vi "Pose2d_NearestTo.vi"(9 "other POSE":T1[](array[typedef]) {"ROTATION"."SIN" format="%13.4f"; "ROTATION"."COS" format="%13.4f"; "ROTATION"."VALUE" format="%13.4f"; "TRANSLATION"."Y" format="%14.3f"; "TRANSLATION"."X" format="%14.3f"}, 11 "in POSE":T1 {"ROTATION"."SIN" format="%13.4f"; "ROTATION"."COS" format="%13.4f"; "ROTATION"."VALUE" format="%13.4f"; "TRANSLATION"."Y" format="%14.3f"; "TRANSLATION"."X" format="%14.3f"}) -> (1 "Found":bool, 3 "Nearest Pose":T1={"TRANSLATION"={"X"=0.0, "Y"=0.0}, "ROTATION"={"VALUE"=0.0, "COS"=1.0, "SIN"=0.0}} {"ROTATION"."SIN" format="%13.4f"; "ROTATION"."COS" format="%13.4f"; "ROTATION"."VALUE" format="%13.4f"; "TRANSLATION"."Y" format="%14.3f"; "TRANSLATION"."X" format="%14.3f"})   [LabVIEW 2019, in "Trajectory_Library.lvlib"]
doc: "Returns the Transform2d that maps the one pose to another.\n\nParameter:\n - IN POSE - Current POSE data structure\n - OTHER POSE - The initial pose of the transformation.\n\nReturns:\n - OUT TRANSFORMATION - The transform that maps the other pose to the current pose."
uses:
  TypeDef/POSE2D.ctl
  TypeDef/TRANSLATION2D.ctl
  TypeDef/ROTATION2D.ctl
  Transform2d_Create_PosePose.vi
  Pose2d_New_TRRO.vi
  Rotation2d_UnaryMinus.vi
  Translation2d_RotateBy.vi
  Translation2d_Minus.vi
  Rotation2d_CreateAngle.vi
  Translation2d_Create.vi
  Rotation2d_RotateBy.vi
  Rotation2d_CreateXY.vi
  Util_CalcDist.vi
  Trajectory_Library.lvlib
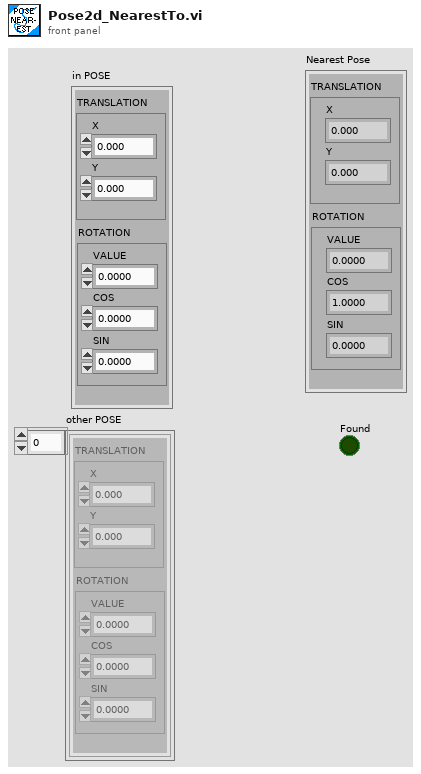
[diagram p1: front panel]
types:
  T1 = typedef "Trajectory_Library.lvlib/POSE2D.ctl" = cluster{"TRANSLATION":T2, "ROTATION":T3}
  T2 = typedef "Trajectory_Library.lvlib/TRANSLATION2D.ctl" = cluster{"X":dbl, "Y":dbl}
  T3 = typedef "Trajectory_Library.lvlib/ROTATION2D.ctl" = cluster{"VALUE":dbl, "COS":dbl, "SIN":dbl}
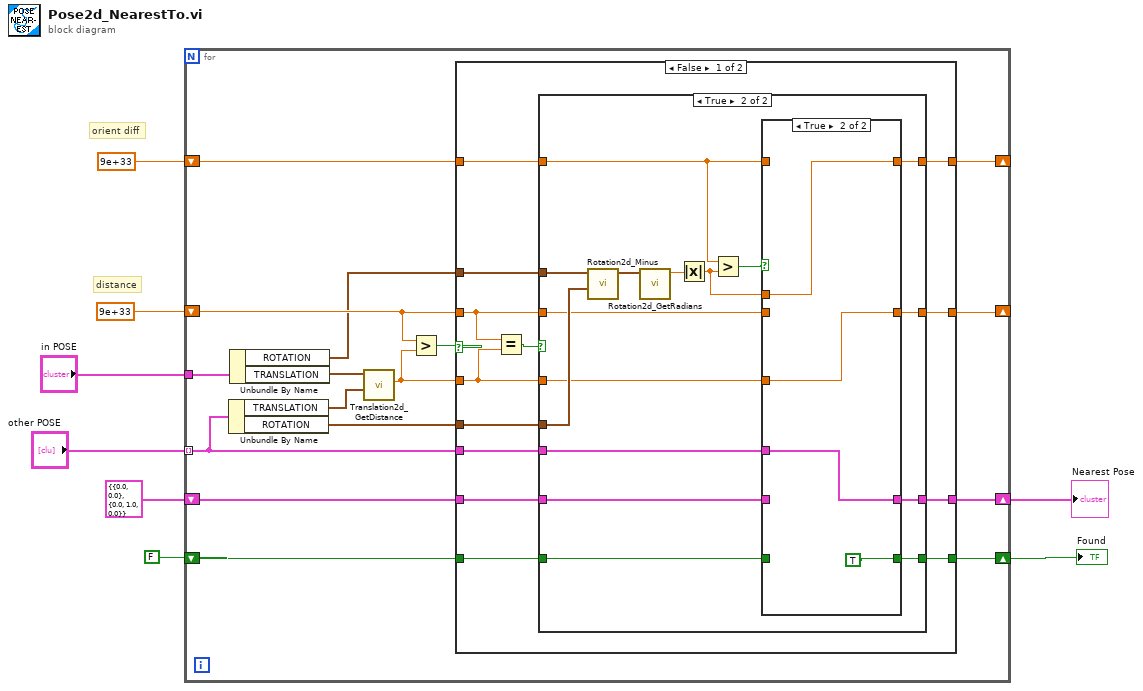
[diagram p0: block diagram]
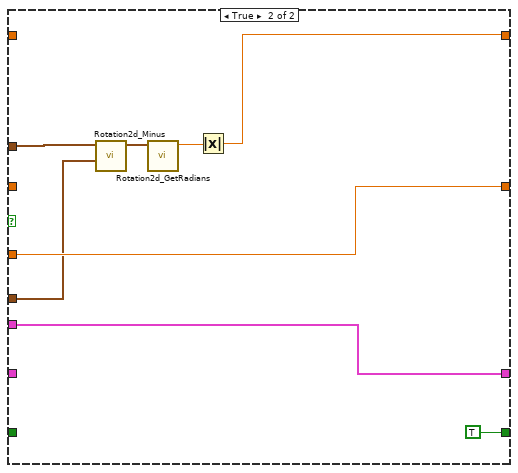
[diagram p4: hidden frame]
diagram:
  # "orient diff"
  # "distance"
  n1 = for {
    shift-right: [w23] -> _
    shift-left: 9e+33 -> [w19]
    tunnel: "in POSE" -> [w16]
    tunnel: "other POSE" -> [w15] mode=indexing
    shift-right: [w20] -> w1
    shift-left: FALSE -> [w17]
    shift-right: [w21] -> w2
    shift-left: T1 {"TRANSLATION"={"X"=0.0, "Y"=0.0}, "ROTATION"={"VALUE"=0.0, "COS"=1.0, "SIN"=0.0}} ("other POSE") -> [w18]
    shift-right: [w11] -> _
    shift-left: 9e+33 -> [w12]
    n2 = Unbundle By Name(w15) -> ("TRANSLATION"=w13:T2, "ROTATION"=w10:T3)
    n3 = Unbundle By Name(w16) -> ("ROTATION"=w9:T3, "TRANSLATION"=w14:T2)
    n4 = call "Translation2d_GetDistance.vi"("other Translation"=w13, "In Translation"=w14) -> ("Distance"=w22:dbl)  [unwired: 9 in]
    n5 = Greater?(x=w19, y=w22) -> (0:w24:bool)
    n6 = case shown="False" w24 {
      tunnel: w15 -> [w25 w72]
      tunnel: [w35 w73] -> w23
      tunnel: w22 -> [w26 w73]
      tunnel: [w32 w72] -> w21
      tunnel: [w31 TRUE] -> w20
      tunnel: w19 -> [w36 _]
      tunnel: w18 -> [w33 _]
      tunnel: w17 -> [w34 _]
      tunnel: w12 -> [w30 _]
      tunnel: [w29 w66] -> w11
      tunnel: w10 -> [w27 w69]
      tunnel: w9 -> [w28 w70]
      frame False {
        n7 = Equal?(x=w36, y=w26) -> (x = y?=w37:bool)
        n8 = case shown="True" w37 {
          tunnel: w36 -> [w41 w44]
          tunnel: [w41 w50] -> w35
          tunnel: w34 -> [w39 w42]
          tunnel: w33 -> [w40 w43]
          tunnel: [w40 w48] -> w32
          tunnel: [w39 w46] -> w31
          tunnel: w30 -> [w38 w45]
          tunnel: [w38 w52] -> w29
          tunnel: w28 -> [_ w55]
          tunnel: w27 -> [_ w54]
          tunnel: w26 -> [_ w49]
          tunnel: w25 -> [_ w47]
          frame False {
          }
          frame True {
            n9 = call "Rotation2d_Minus.vi"("other ROTATION"=w54, "in ROTATION"=w55) -> ("out ROTATION"=w57:T3)  [unwired: 9 in]
            n10 = call "Rotation2d_GetRadians.vi"("in ROTATION"=w57) -> ("AngleRadians"=w56:dbl)  [unwired: 10 in]
            n11 = Absolute Value(x=w56) -> (abs(x)=w51:dbl)
            n12 = Greater?(x=w45, y=w51) -> (0:w53:bool)
            n13 = case shown="True" w53 {
              tunnel: [w61 w65] -> w52
              tunnel: w51 -> [_ w65]
              tunnel: [w60 w64] -> w50
              tunnel: w49 -> [_ w64]
              tunnel: [w59 w63] -> w48
              tunnel: w47 -> [_ w63]
              tunnel: [w58 TRUE] -> w46
              tunnel: w45 -> [w61 _]
              tunnel: w44 -> [w60 _]
              tunnel: w43 -> [w59 _]
              tunnel: w42 -> [w58 _]
              frame False {
              }
              frame True {
              }
            }
          }
        }
      }
      frame True {
        n14 = call "Rotation2d_Minus.vi"("other ROTATION"=w69, "in ROTATION"=w70) -> ("out ROTATION"=w68:T3)  [unwired: 9 in]
        n15 = call "Rotation2d_GetRadians.vi"("in ROTATION"=w68) -> ("AngleRadians"=w67:dbl)  [unwired: 10 in]
        n16 = Absolute Value(x=w67) -> (abs(x)=w66:dbl)
      }
    }
  }
  "Nearest Pose" <- w2
  "Found" <- w1
